vi "Sound TEsting.vi"() -> ()   [LabVIEW 2013]
uses:
  <vilib>/LabVIEW Interface for Arduino/Type Defs/Board Type.ctl
  <vilib>/LabVIEW Interface for Arduino/Type Defs/Connection Type.ctl
  <vilib>/LabVIEW Interface for Arduino/LabVIEW Interface for Arduino.lvlib
panel:
  out "millisec":dbl
  out "millisec":dbl
  out "Hz":dbl
  in  "Delay":dbl(knob) scale=0.0..10000.0
  in  "stop":bool
  in  "Duration":dbl(knob) scale=0.0..1000.0
  in  "Frequency":dbl(knob) min=0.0 max=20000.0 step=0.5 scale=0.0..30000.0
  in  "Tone DO Pin":u8=8
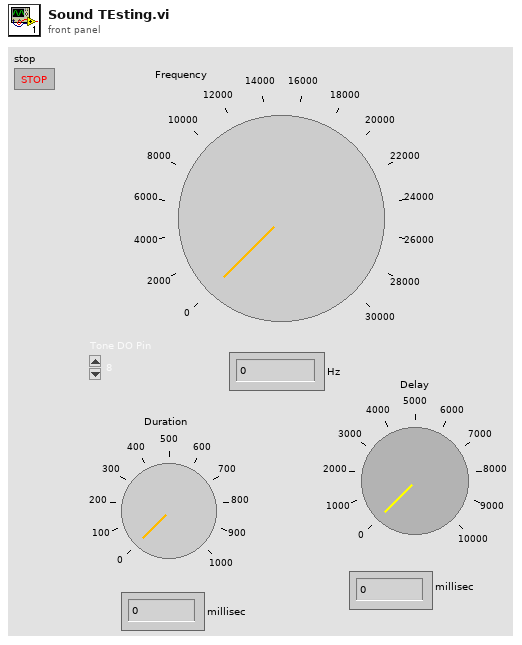
[diagram p1: front panel]
types:
  T1 = typedef "LabVIEW Interface for Arduino.lvlib/Connection Type.ctl" = enum8{"USB / Serial", "XBEE", "BlueSmirf (Bluetooth)"}
  T2 = typedef "LabVIEW Interface for Arduino.lvlib/Board Type.ctl" = enum16{"Uno", "Dimuelanove w/Atmega 328", "Mega 2560"}
  T3 = typedef "LabVIEW Interface for Arduino.lvlib/Arduino Resource.ctl" = cluster{"VISA resource":refnum<visa-resource-name>, "Board Type":T2, "Connection Type":enum8{"USB / Serial"}, "Bytes Per Packet (15)":u8}
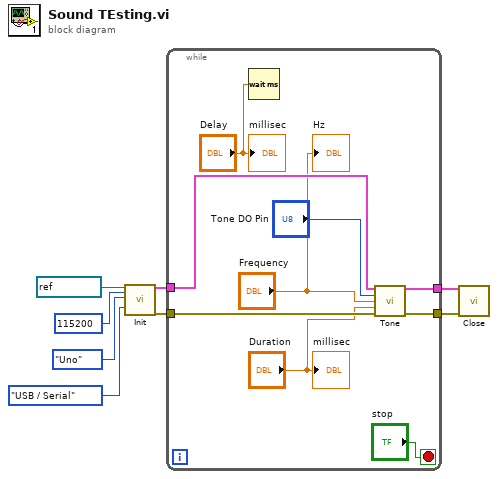
[diagram p0: block diagram]
diagram:
  n1 = call <vilib>:"Init.vi"("VISA resource"=refnum<visa-resource-name> "COM5", "Baud Rate (115200)"=u32 115200, "Board Type (Uno)"=Board_Type."Uno", "Connection Type (USB/Serial)"=Connection_Type."USB / Serial") -> ("Arduino Resource"=w8:T3, "error out"=w6:errorcluster)  [unwired: 14 in]
  n2 = while {
    tunnel: w8 -> [w17]
    tunnel: [w16] -> w7
    tunnel: w6 -> [w15]
    tunnel: [w14] -> w5
    stop <- "stop" stop-if-true
    n3 = Wait (ms)(milliseconds to wait="Delay") -> ()  [unwired: 1 out]
    n4 = call <vilib>:"Tone.vi"("Arduino Resource"=w17, "Tone DO Pin"="Tone DO Pin", "Frequency (0 Hz)"="Frequency", "Duration (1 ms)"="Duration", "error in"=w15) -> ("Arduino Resource"=w16:T3, "error out"=w14:errorcluster)  [unwired: 9 in]
    "Hz" <- "Frequency"
    "millisec" <- "Duration"
    "millisec" <- "Delay"
  }
  n5 = call <vilib>:"Close.vi"("Arduino Resource"=w7, "error in"=w5) -> ()  [unwired: 13 in, 1 out]
